vi "Channel Properties.vi"(8 "error in (no error)":errorcluster, 10 "Channel Settings Ref In":refnum<vi>, 11 "Channel Ref In":T1 format="%.0x") -> (0 "error out":errorcluster, 3 "Channel Ref Out":T1 format="%.0x")   [LabVIEW 2015, in "DMM-SWITCH-ScanList System Explorer.lvlib"]
uses:
  DMM-SWITCH-ScanList System Explorer.lvlib
  <vilib>/NI Veristand/Custom Device API/Custom Device Item Ref.ctl
  <vilib>/NI Veristand/Custom Device API/Custom Device API.lvlib
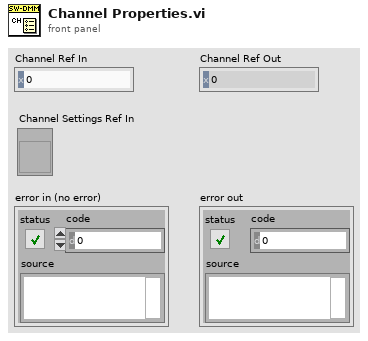
[diagram p1: front panel]
types:
  T1 = typedef "Custom Device API.lvlib/Custom Device Item Ref.ctl" = u64
  T2 = typedef "Custom Device API.lvlib/Custom Device Channel.ctl" = cluster{"Type":T3, "Units":string, "Default Value":dbl, "Faultable":bool, "Scalable":bool}
  T3 = typedef "Custom Device API.lvlib/Custom Device Channel Type.ctl" = enum16{"Input", "Output"}
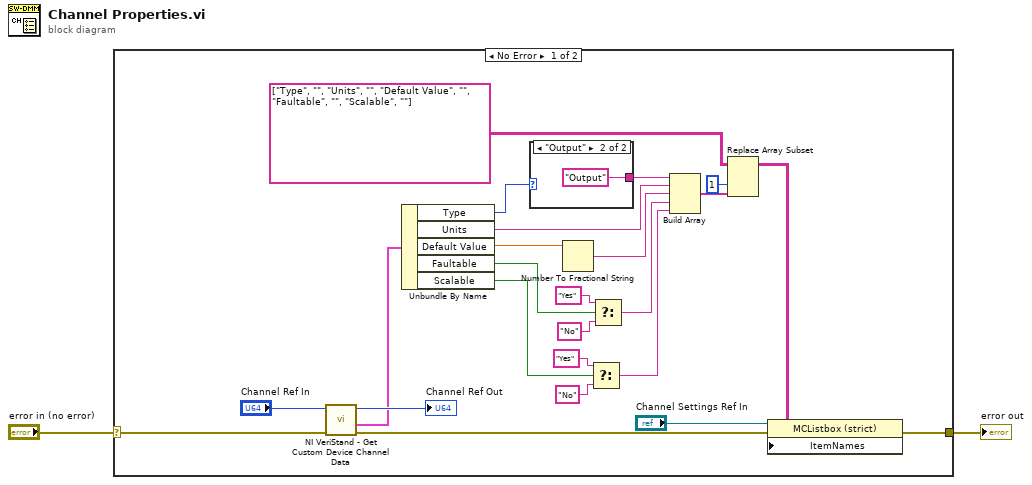
[diagram p0: block diagram]
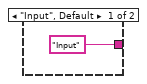
[diagram p2: hidden frame]
diagram:
  n1 = case shown="No Error" "error in (no error)" {
    selector: "error in (no error)" -> [w3 w29]
    tunnel: [w26 w29] -> w2
    frame No Error {
      n2 = call <vilib>:"NI VeriStand - Get Custom Device Channel Data.vi"("error in (no error)"=w3, "Channel Ref in"="Channel Ref In") -> ("error out"=w25:errorcluster, "Channel"=w5:T2, "Channel Ref out"=→"Channel Ref Out":T1)  [unwired: 4 in, 3 out]
      n3 = Unbundle By Name(w5) -> ("Type"=w8:T3, "Units"=w10:string, "Default Value"=w11:dbl, "Faultable"=w13:bool, "Scalable"=w19:bool)
      n4 = case shown="\"Output\"" w8 {
        tunnel: ["Input" "Output"] -> w9
        frame "Input", Default {
        }
        frame "Output" {
        }
      }
      n5 = Number To Fractional String(number=w11) -> (F-format string=w12:string)  [unwired: 3 in]
      n6 = Select(t="Yes", s=w19, f="No") -> (s? t:f=w20:string)
      n7 = Select(t="Yes", s=w13, f="No") -> (s? t:f=w16:string)
      n8 = Build Array(w9, w10, w12, w16, w20) -> (w22:string[])
      n9 = Replace Array Subset(array=string[][] [["Type", ""], ["Units", ""], ["Default Value", ""], ["Faultable", ""], ["Scalable", ""]] ("Item Names"), new element=w22, index (col)=1 ("disabled index (col)")) -> (w24:string[][])  [unwired: 1 in]
      n10 = property on="Property Node" class="MCListbox (strict)"(reference="Channel Settings Ref In", error in=w25, "ItemNames"=w24) -> (error out=w26:errorcluster)  [unwired: 1 out]
    }
    frame Error {
    }
  }
  "error out" <- w2
